vi "Recursive Model&Adaptive Control.vi"() -> ()   [LabVIEW 2015]
uses:
  <vilib>/addons/Control Design/_Model Construction/Model Typedefs.llb/CD State Space Model (MIMO).ctl
  <vilib>/addons/Control Design/_Model Construction/Model Typedefs.llb/CD General Elements.ctl
  <vilib>/Platform/TimedLoop/XDataNode/timing_clust.ctl
  <vilib>/Platform/TimedLoop/XDataNode/nitl_modes.ctl
  <vilib>/Platform/TimedLoop/XDataNode/wakeup.ctl
  <vilib>/FPGAPlugInAG/myRIO-1900/niLvFpga_Open_myRIO-1900.vi
  <vilib>/rvi/interface/common/dynamic/niFpgaDynamicAddResources.vi
  <vilib>/Utility/error.llb/Error Cluster From Error Code.vi
  <vilib>/rvi/errors/niLvFpgaAdjustHostInterfaceError.vi
  <vilib>/FPGAPlugInAG/Dynamic/niLvFpga_Close_Dynamic.vi
  <vilib>/Analysis/7linalg.llb/Create Special Real Matrix.vi
  <vilib>/addons/Control Design/_Model Construction/Model Creation.llb/Model Creation SubVI/cd_Create State Space Model.vi
  <vilib>/addons/Control Design/_Stochastic Systems/Stochastic Systems.llb/CD Construct Noise Model (Numeric).vi
  <vilib>/addons/Control Design/_State Feedback Control/State Feedback Control.llb/State Feedback Control SubVis/cd_Discretized Linear Quadratic Regulator.vi
  <vilib>/Simulation/Estimation/Implementation/NILVSim Discrete Kalman Filter.llb/SIM Disc KF Pred and Corr with Pred Gain with Checking Direct LV.vi
  <vilib>/rvi/interface/nirviOpenFPGA/nirviOpenFPGA.xnode
  FPGA Bitfiles/ACC20115_FPGATarget_CurrentControlle_Dt5vFgOzYtY.lvbitx
  Current Controller.vi
  <vilib>/rvi/interface/nirviReadWriteControl/nirviReadWriteControl.xnode
  <vilib>/rvi/interface/nirviCloseFPGA/nirviCloseFPGA.xnode
  <vilib>/Platform/TimedLoop/XDataNode/XDataNode.xnode
  <vilib>/Simulation/Implementation/XNodeFramework/SimXNode/SimX.xnode
  NiFpgaLv.dll
  <vilib>/rvi/interface/Simulation/niFpgaSimulationCallBeginRW.vi
  <vilib>/addons/Control Design/_State Feedback Control/NI_CD_State Feedback Control.lvlib
  <vilib>/addons/Control Design/_Stochastic Systems/NI_CD_Stochastic Systems.lvlib
  <vilib>/Platform/TimedLoop/XDataNode/XDNodeRunTimeDep.lvlib
  <vilib>/Analysis/NI_AALPro.lvlib
  <vilib>/addons/Control Design/_Model Construction/NI_LinSys_Model Creation.lvlib
  <vilib>/addons/Control Design/_State-Space Analysis/NI_CD_State-Space Analysis.lvlib
  <vilib>/addons/Control Design/_Model Construction/NI_LinSys_Model Typedefs.lvlib
panel:
  out "error IO":errorcluster
  out "KF Predictor Gain L(k)":dbl[][](array[numeric])
  out "KF Gain M(k)":dbl[][](array[numeric])
  out "xhat(k+1|k)":dbl[](array[numeric])
  out "xhat(k|k)":dbl[](array[numeric])
  in  "Tab Control":enum32{"Outputs/Control", "Model Info"}(tab)
  out "DAC Inlet Valve 2":i32(graph)
  out "Fusion Data":dbl(graph)
  in  "SP1:":dbl(slide)=40.87020302841148 min=0.0 max=0.0 scale=0.0..720.0
  in  "Stop":bool
  out "FPGA Status?":bool
  in  "Current (mA)":i32
  out "Priori SS Detectable?":bool
  out "Priori SS Observable?":bool
  out "KF estimate":dbl[](graph)
  out "State-Space Model":T1 {"Transport Delay" format="%.2f"; "D" format="%#.2g"; "C" format="%#.2g"; "B" format="%#.2g"; "A" format="%#.2g"; "properties"."Sampling Time" format="%#.6p"; "properties"."Output Delays" format="%.4f"; "properties"."Input Delays" format="%.4f"}
  in  "LQR State Weight Matrix (Q)":dbl[](array[slide])=[1.133823501217849, 15.19911082952933] scale=0.001..1000.0
  in  "LQR Output weighting matrix (R)":dbl[](array[slide])=[0.061359072734131735] scale=0.0001..10.0
  in  "A":dbl[][](array[numeric]) format="%#.5g"
  in  "B":dbl[][](array[numeric]) format="%#.5g"
  in  "C":dbl[][](array[numeric]) format="%#.5g"
  in  "D":dbl[][](array[numeric]) format="%#.5g"
  in  "KF P(0|-1)":dbl[][](array[numeric])=[[1.0]]
  in  "xhat(0|-1)":dbl[](array[numeric])=[1.0]
  in  "E{w}":dbl[](array[numeric]) format="%#.2g"
  in  "E{v}":dbl[](array[numeric]) format="%#.2g"
  in  "KF R":dbl[][](array[numeric]) format="%#.2g"
  in  "KF Q":dbl[][](array[numeric]) format="%#.2g"
  in  "G":dbl[][](array[numeric]) format="%#.2g"
  in  "H":dbl[][](array[numeric]) format="%#.2g"
  in  "N":dbl[][](array[numeric]) format="%.2f"
  out "Riccati Solution (X)":dbl[][](array[numeric]) format="%.4f"
  out "error out":errorcluster
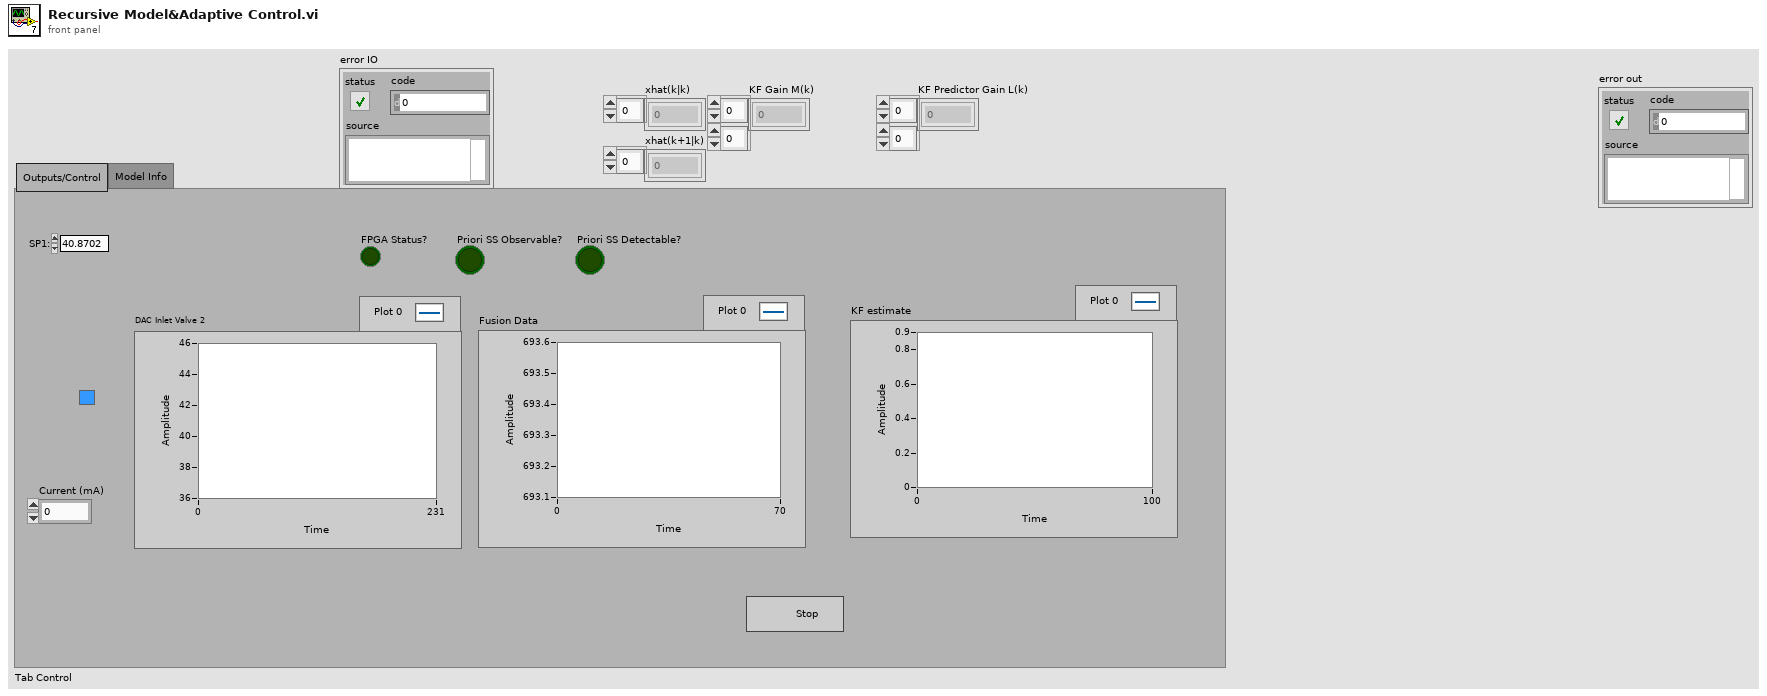
[diagram p1: front panel]
types:
  T1 = typedef "NI_LinSys_Model Typedefs.lvlib/CD State Space Model (MIMO).ctl" = cluster{"properties":T2, "A":dbl[][], "B":dbl[][], "C":dbl[][], "D":dbl[][], "StateNames":string[], "Transport Delay":dbl[][]}
  T2 = typedef "NI_LinSys_Model Typedefs.lvlib/CD General Elements.ctl" = cluster{"Model name":string, "Input names":string[], "Output names":string[], "Input Delays":dbl[], "Output Delays":dbl[], "Sampling Time":dbl, "Notes":string}
  T3 = typedef "XDNodeRunTimeDep.lvlib/timing_clust.ctl" = cluster{"Expected End [f-1]":u64, "Actual End [f-1]":u64, "Finished Late? [f-1]":bool, "Expected End [i-1]":u64, "Actual End [i-1]":u64, "Finished Late? [i-1]":bool, "Expected Start [i]":u64, "Actual Start [i]":u64, "Expected Start [f]":u64, "Actual Start [f]":u64, "Source Name":string, "Structure Name":string, "Period":i64, "Deadline":i64, "Offset":i64, "Start":i64, "Priority":i32, "Timeout":i32, "Mode":T4, "Wakeup Reason":T5, "Error":errorcluster, "Source Type":string, "Secondary Source Type":string, "Global End Time":u64, "Global Start Time":u64, "Frame Duration":u64, "Iteration Duration":u64, "Assigned CPU":i32, "I/O Scan Engine Mode":u32}
  T4 = typedef "XDNodeRunTimeDep.lvlib/nitl_modes.ctl" = enum32{"No Change", "Process missed periods, maintain original phase", "Discard missed periods, maintain original phase", "Process missed periods, ignore original phase", "Discard missed periods, ignore original phase"}
  T5 = typedef "XDNodeRunTimeDep.lvlib/wakeup.ctl" = enum32{"Normal", "Aborted", "Asynchronous wakeup", "Timing source error", "Timed loop error", "Timeout"}
  T6 = enum16{"state weighting", "output weighting, Dim Q = Ny", "output weighting, Dim Q = Nx"}
  T7 = enum32{"Identity", "Diagonal", "Toepliz", "Vandermonde", "Companion"}
  T8 = typedef "NI_CD_Stochastic Systems.lvlib/cd_Stochastic State-Space Model.ctl" = cluster{"Sampling Time (s)":dbl, "G":dbl[][], "B":dbl[][], "A":dbl[][], "C":dbl[][], "D":dbl[][], "H":dbl[][]}
  T9 = typedef "NI_Matrix.lvlib/RealMatrix.ctl" = dbl[][]
  T10 = typedef "NI_CD_Stochastic Systems.lvlib/cd_Second-Order Statistics Noise Model.ctl" = cluster{"Q":dbl[][], "E{w}":dbl[], "E{v}":dbl[], "R":dbl[][], "N":dbl[][]}
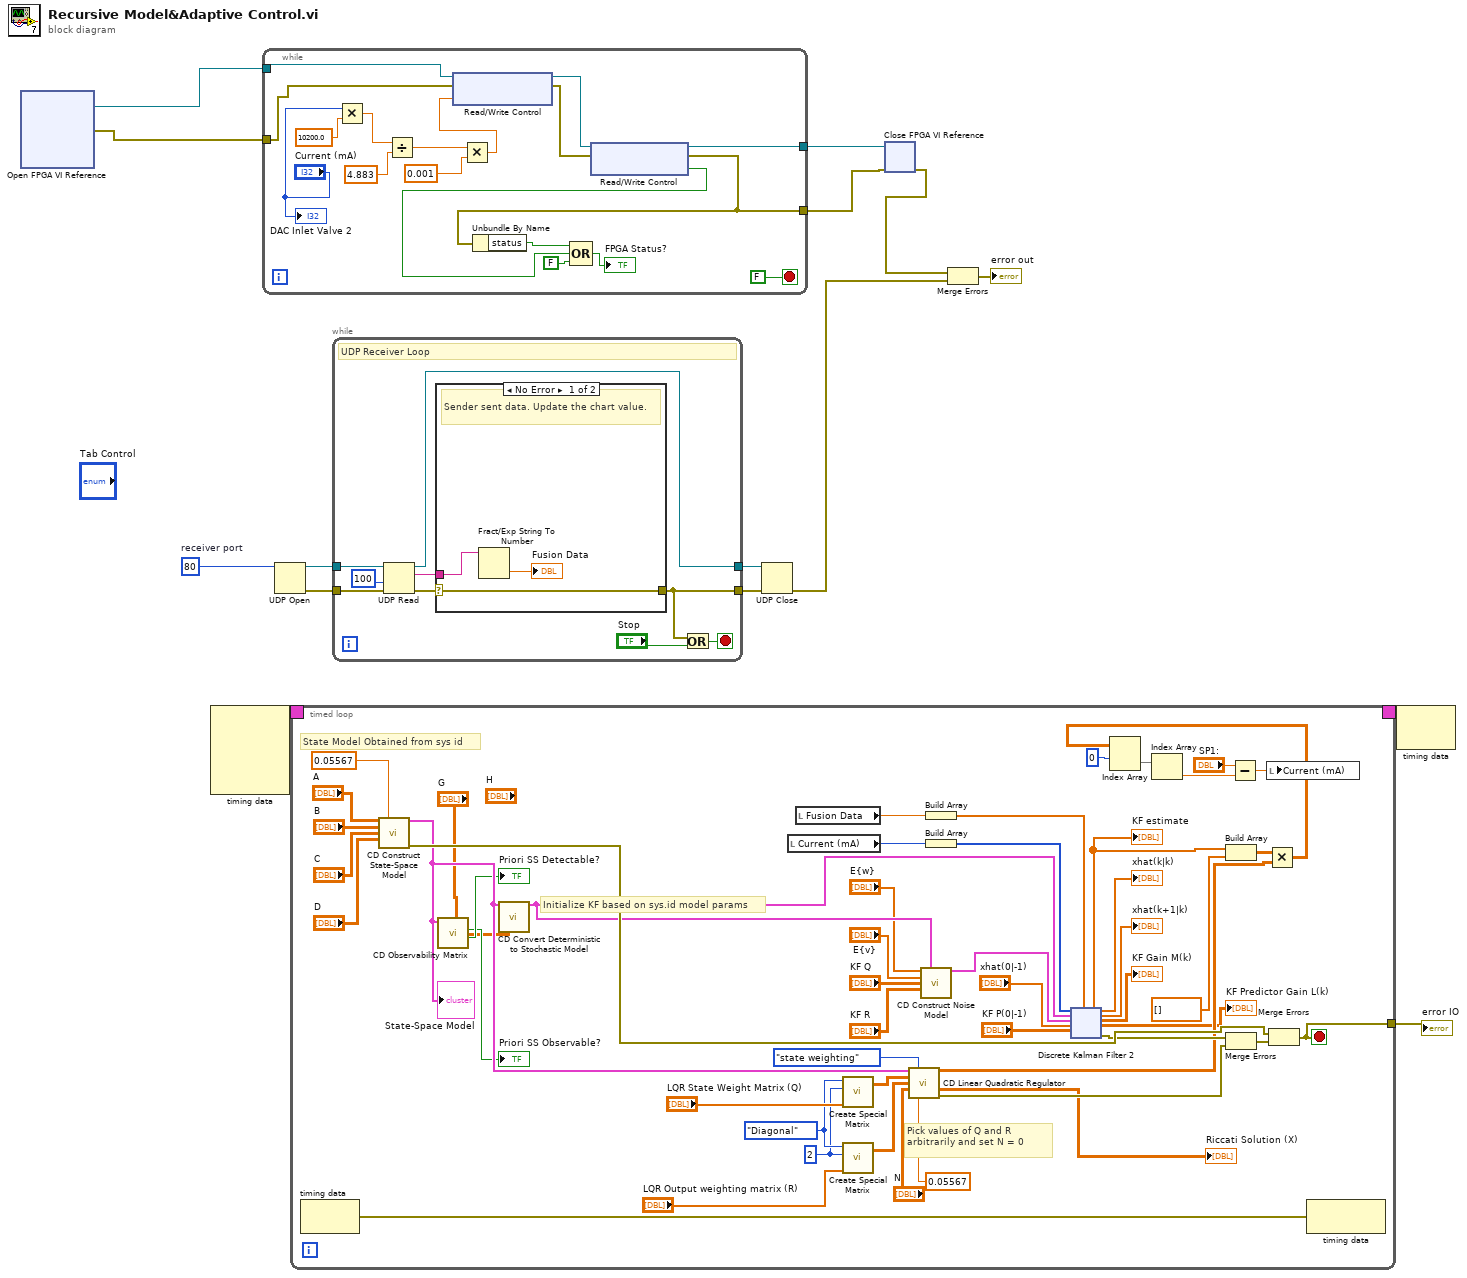
[diagram p0: block diagram]
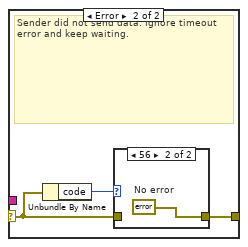
[diagram p2: hidden frame]
diagram:
  w11 = u16 80  # receiver port
  n1 = xnode "Open FPGA VI Reference"() -> ("FPGA VI Reference Out"=w4:refnum<k20>, "error out"=w5:errorcluster)  [unwired: 2 in]
  n2 = node-c288() -> (w3:T3)  [unwired: 4 in]
  n3 = while {
    tunnel: w4 -> [w32]
    tunnel: w5 -> [w16]
    tunnel: [w26] -> w9
    tunnel: [w24] -> w10
    stop <- FALSE stop-if-true
    n4 = Multiply(x="Current (mA)", y=10200.0) -> (x*y=w19:dbl)
    n5 = Divide(x=w19, y=4.883) -> (x/y=w22:dbl)
    n6 = Multiply(x=w22, y=0.001) -> (x*y=w18:dbl)
    n7 = xnode "Read/Write Control"("FPGA VI Reference In"=w32, "error in"=w16, "DAC Inlet Valve"=w18) -> ("FPGA VI Reference Out"=w31:refnum<k20>, "error out"=w30:errorcluster)
    n8 = xnode "Read/Write Control"("FPGA VI Reference In"=w31, "error in"=w30) -> ("FPGA VI Reference Out"=w24:refnum<k20>, "error out"=w26:errorcluster, "Inlet Overflow?"=w25:bool)
    n9 = Unbundle By Name(w26) -> ("status"=w28:bool)
    n10 = Compound Arithmetic op=OR(w28, w25, FALSE ("value")) -> (→"FPGA Status?":bool)
    "DAC Inlet Valve 2" <- "Current (mA)"
  }
  n11 = UDP Open(11:w11) -> (port=w12:refnum<k16>, 0:w13:errorcluster)  [unwired: 4 in, 1 out]
  n12 = timed-loop {
    tunnel: [w57] -> w1
    timing: w3 -> [_]
    timing-out: [_] -> w2
    stop <- w57 stop-if-true
    w58 = 2
    w64 = T7."Diagonal" ("matrix type")
    # "Pick values of Q and R\narbitrarily and set N = 0"
    # "State Model Obtained from sys id"
    # "Initialize KF based on sys.id model params"
    n13 = node-c288() -> (w56:errorcluster)  [unwired: 1 in]
    n14 = call-poly <vilib>:"CD Construct State-Space Model.vi"("A"="A", "Sampling Time (s)"=0.05567, "B"="B", "C"="C", "D"="D") -> ("State-Space Model"=w49:T1, "error out"=w72:errorcluster)  [unwired: 9 in]
    "State-Space Model" <- w49
    n15 = call <vilib>:"CD Observability Matrix.vi"("State-Space Model"=w49) -> ("Is Detectable?"=→"Priori SS Detectable?":bool, "Is Observable?"=→"Priori SS Observable?":bool)  [unwired: 7 in, 2 out]
    n16 = call <vilib>:"CD Convert Deterministic to Stochastic Model.vi"("Deterministic State-Space Model"=w49, "G"="G") -> ("Stochastic State-Space Model"=w68:T8)  [unwired: 12 in, 1 out]
    n17 = local read "Current (mA)"() -> (w73:i32)
    n18 = local read "Fusion Data"() -> (w75:dbl)
    n19 = call-poly <vilib>:"Create Special Matrix.vi"("matrix type"=w64, "matrix size"=w58, "Input Vector1"="LQR State Weight Matrix (Q)") -> ("Special Matrix"=w62:T9)  [unwired: 2 in, 1 out]
    n20 = call-poly <vilib>:"Create Special Matrix.vi"("matrix type"=w64, "matrix size"=w58, "Input Vector1"="LQR Output weighting matrix (R)") -> ("Special Matrix"=w61:T9)  [unwired: 2 in, 1 out]
    n21 = call-poly <vilib>:"CD Linear Quadratic Regulator.vi"("Continuous State-Space Model"=w49, "Weighting Type"=T6."state weighting", "Q"=w62, "R"=w61, "N"="N", "Sampling Time (s)"=0.05567) -> ("Optimal Gain (K)"=w60:dbl[][], "Riccati Solution (X)"=→"Riccati Solution (X)":dbl[][], "error out"=w59:errorcluster)  [unwired: 6 in, 1 out]
    n22 = call-poly <vilib>:"CD Construct Noise Model.vi"("E{w}"="E{w}", "Stochastic State-Space Model"=w68, "E{v}"="E{v}", "Q"="KF Q", "R"="KF R") -> ("Second-Order Statistics Noise Model out"=w42:T10)  [unwired: 9 in, 1 out]
    n23 = Build Array ("Build Array 6")(w75) -> (w71:dbl[])
    n24 = Build Array ("Build Array 5")(w73) -> (w67:i32[])
    n25 = xnode ("Discrete Kalman Filter 2")("input u(k)"=w67, "Stochastic State-Space Model"=w68, "Second-Order Statistics Noise Model"=w42, "Initial State Estimate xhat(0|-1)"="xhat(0|-1)", "Initial Estimation Error Covariance P(0|-1)"="KF P(0|-1)", "Output y(k)"=w71) -> ("Estimated Output yhat(k)"=w70:dbl[], "Corrected State Estimate xhat(k|k)"=→"xhat(k|k)":dbl[], "Predicted State Estimate xhat(k+1|k)"=→"xhat(k+1|k)":dbl[], "Kalman Filter Gain M(k)"=→"KF Gain M(k)":dbl[][], "Kalman Predictor Gain L(k)"=→"KF Predictor Gain L(k)":dbl[][], "error out"=w69:errorcluster)  [unwired: 2 in, 2 out]
    "KF estimate" <- w70
    n26 = Build Array ("Build Array 9")(w70, dbl[] [] ("element")) -> (w80:dbl[][])
    n27 = Merge Errors(w69, w59) -> (w78:errorcluster)
    n28 = Multiply(x=w80, y=w60) -> (x*y=w82:dbl[][])
    n29 = Index Array(array=w82, index (row)=0) -> (element=w84:dbl[])  [unwired: 1 in]
    n30 = Index Array ("Index Array 2")(array=w84) -> (element=w76:dbl)  [unwired: 1 in]
    n31 = Subtract(x="SP1:", y=w76) -> (x-y=w74:dbl)
    n32 = local write "Current (mA)"(w74) -> ()
    n33 = Merge Errors(w72, w78) -> (w57:errorcluster)
    n34 = node-c288(w56) -> ()  [unwired: 1 out]
  }
  "error IO" <- w1
  n35 = while {
    tunnel: w12 -> [w114]
    tunnel: [w106] -> w15
    tunnel: w13 -> [w111]
    tunnel: [w107] -> w14
    stop <- w112 stop-if-true
    # "UDP Receiver Loop"
    n36 = UDP Read(connection ID=w114, timeout ms (25000)=100, 8:w111) -> (data out=w109:string, error out=w108:errorcluster, 3:w106:refnum<k16>)  [unwired: 3 out]
    n37 = case shown="No Error" w108 {
      selector: w108 -> [w115 w119]
      tunnel: w109 -> [w117 _]
      tunnel: [w115 w118] -> w107
      frame No Error {
        # "Sender sent data. Update the chart value."
        n38 = Fract/Exp String To Number(string=w117) -> (number=→"Fusion Data":dbl)  [unwired: 3 in, 1 out]
      }
      frame Error {
        # "Sender did not send data. Ignore timeout error and keep waiting."
        n39 = Unbundle By Name(w119) -> ("code"=w120:i32)
        n40 = case shown="56" w120 {
          tunnel: w119 -> [w121 _]
          tunnel: [w121 w122] -> w118
          frame Default {
          }
          frame 56 {
            w122 = errorcluster {"status"=FALSE, "code"=0, "source"=""}  # No error
          }
        }
      }
    }
    n41 = Or(x=w107, y="Stop") -> (x .or. y?=w112:bool)
  }
  n42 = UDP Close(connection ID=w15, 8:w14) -> (error out=w7:errorcluster)  [unwired: 1 out]
  n43 = xnode "Close FPGA VI Reference"("FPGA VI Reference In"=w10, "error in"=w9) -> ("error out"=w8:errorcluster)
  n44 = Merge Errors(w8, w7) -> (→"error out":errorcluster)
  n45 = node-c288(w2) -> ()  [unwired: 1 out]
